vi "Start Sync.vi"(8 "error in":errorcluster, 11 "ServiceBase out":refnum<class "ServiceBase.lvclass">) -> (0 "error out":errorcluster, 3 "ServiceBase out":refnum<class "ServiceBase.lvclass">)   [LabVIEW 2024, in "gRPC-servicer.lvlib" / "ServiceBase.lvclass"]
uses:
  ServiceBase.lvclass
  ServiceBase.lvclass/ServiceBase.ctl
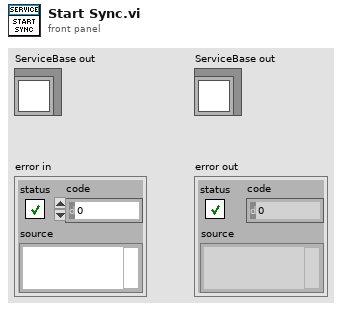
[diagram p1: front panel]
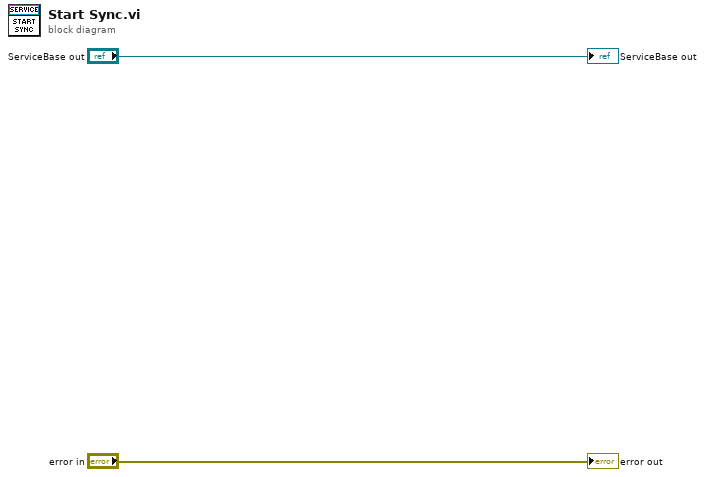
[diagram p0: block diagram]
diagram:
  "error out" <- "error in"
  "ServiceBase out" <- "ServiceBase out"
